vi "Instrument.logToDatabase.vi"(8 "error in (no error)":errorcluster, 9 "Data":variant=variant(bool FALSE), 10 "Paths":string, 11 "Instrument":refnum<class "Instrument.lvclass">) -> (0 "error out":errorcluster, 3 "Instrument out":refnum<class "Instrument.lvclass">)   [LabVIEW 2019, in "Instrument.lvlib" / "Instrument.lvclass"]
doc: "Log data to database\n<b>Paths</b> is a path or list of paths\n<b>Data</b> object containing data to log, typically contained in a cluster if logging multiple items"
uses:
  Instrument.lvclass
  Typedefs/PrivateEvents--Instrument.LogData.ctl
panel:
  # "For instructions on how to use the JKI State Machine Objects, examples and video tutorials, visit:\nhttp://jki.net/state-machine-objects/\n\nJKI State Machine Objects™\nhttp://jki.net/state-machine-objects/\nCopyright (C) 2005-2015, JKI <info@jki.net>\nALL RIGHTS RESERVED"
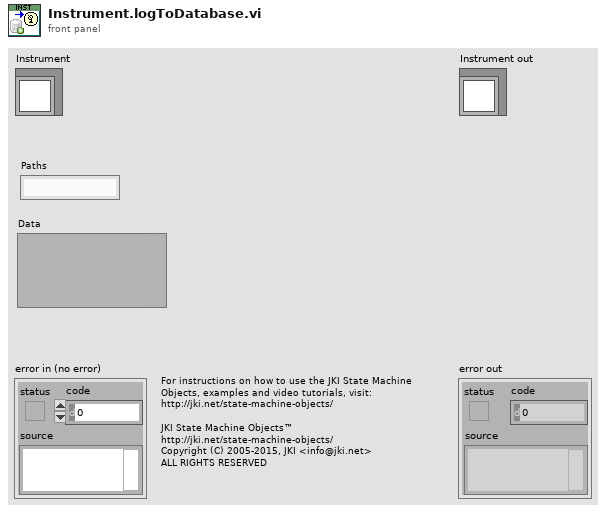
[diagram p1: front panel]
types:
  T1 = typedef "Instrument.lvlib/Instrument.lvclass/PrivateEvents--Instrument.LogData.ctl" = cluster{"path":string, "Data":variant}
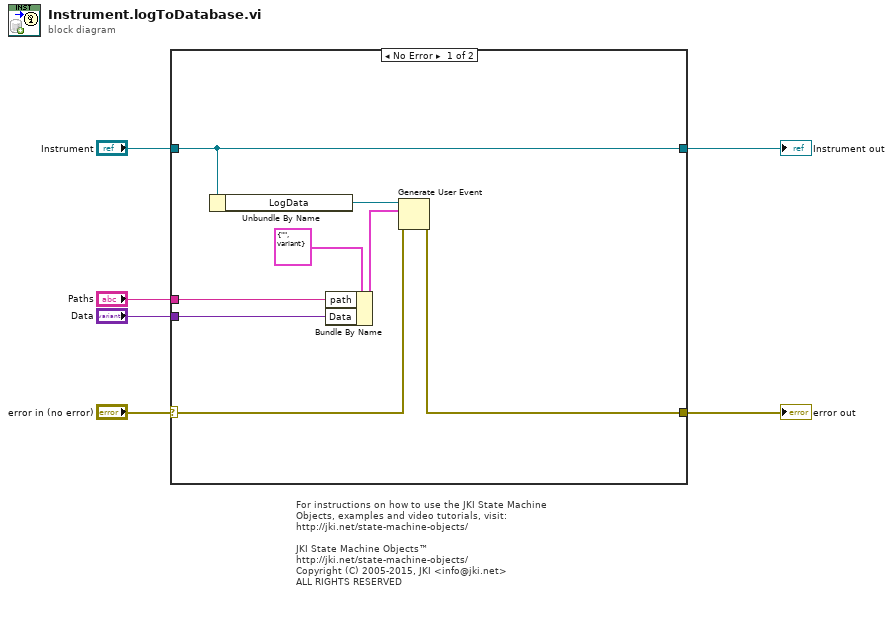
[diagram p0: block diagram]
diagram:
  # "For instructions on how to use the JKI State Machine Objects, examples and video tutorials, visit:\nhttp://jki.net/state-machine-objects/\n\nJKI State Machine Objects™\nhttp://jki.net/state-machine-objects/\nCopyright (C) 2005-2015, JKI <info@jki.net>\nALL RIGHTS RESERVED"
  n1 = case shown="No Error" "error in (no error)" {
    selector: "error in (no error)" -> [w14 w16]
    tunnel: [w12 w16] -> w5
    tunnel: [w11 w15] -> w6
    tunnel: "Instrument" -> [w11 w15]
    tunnel: "Paths" -> [w8 _]
    tunnel: "Data" -> [w7 _]
    frame No Error {
      n2 = Unbundle By Name(w11) -> ("LogData"=w13:refnum<user-event>)
      n3 = Bundle By Name(cluster=T1 {"path"="", "Data"=variant(bool FALSE)} ("Log PGSQL"), "path"=w8, "Data"=w7) -> (w9:T1)
      n4 = Generate User Event(user event=w13, event data cluster=w9, error in=w14) -> (error out=w12:errorcluster)  [unwired: 1 in, 1 out]
    }
    frame Error {
    }
  }
  "error out" <- w5
  "Instrument out" <- w6
